vi "GPS data to cluster.vi"(2 "Speed Threshold (km/h)":dbl, 3 "Gps raw data in":string) -> (0 "Arm System?":bool, 1 "GPS Cluster":cluster{"Lat":dbl, "Lon":dbl, "Speed":dbl})   [LabVIEW 2020]
uses:
  <vilib>/express/express arith-compare/Formula/XNode/ExpressFormulaBlockNode.xnode
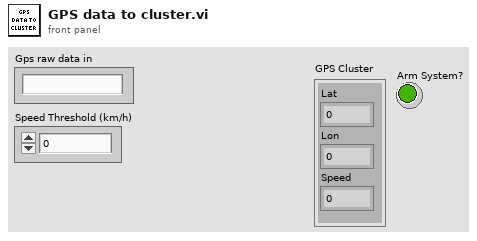
[diagram p1: front panel]
types:
  T1 = typedef "LVDateTimeRec.ctl" = cluster{"fractional second":dbl, "second":i32, "minute":i32, "hour":i32, "day of month":i32, "month":i32, "year":i32, "day of week":i32, "day of year":i32, "DST":i32}
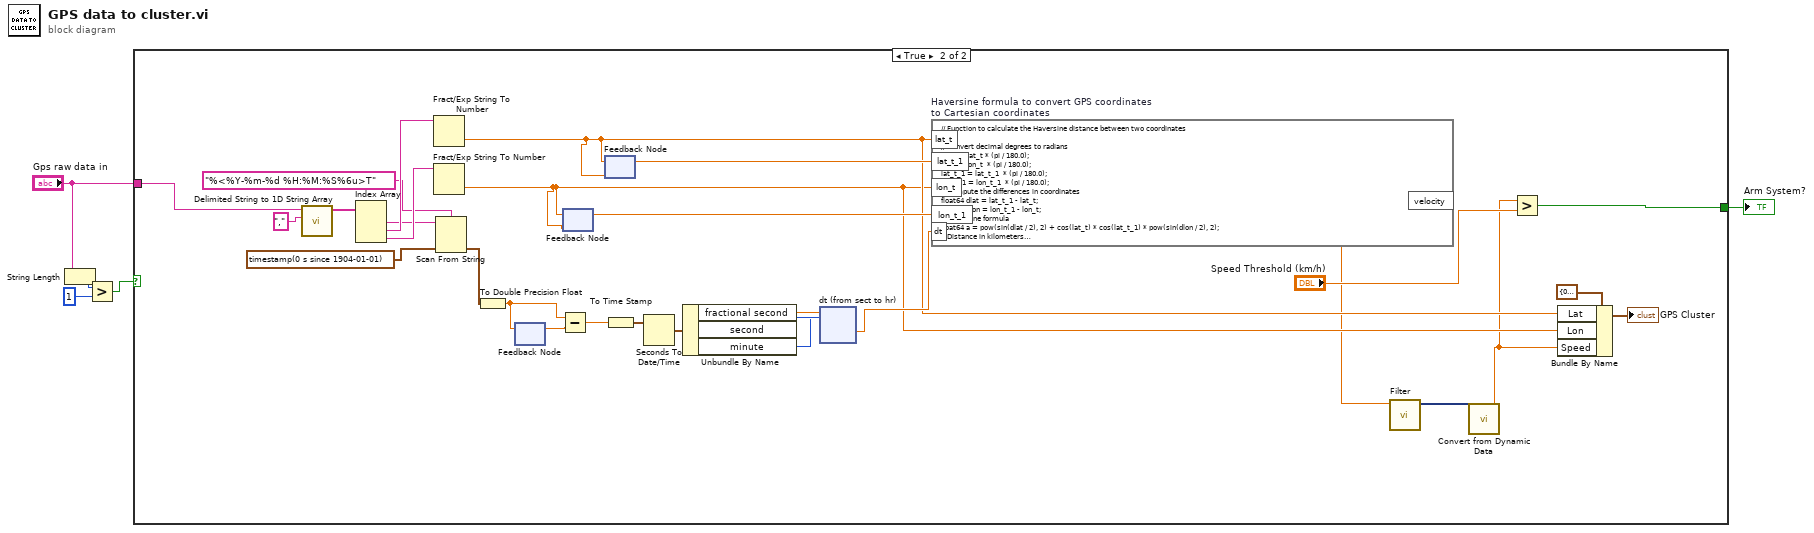
[diagram p0: block diagram]
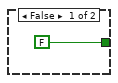
[diagram p2: hidden frame]
diagram:
  n1 = String Length(string="Gps raw data in") -> (length=w2:i32)
  n2 = Greater?(x=w2, y=1) -> (0:w3:bool)
  n3 = case shown="True" w3 {
    tunnel: "Gps raw data in" -> [_ w18]
    tunnel: [FALSE w15] -> w5
    frame False {
    }
    frame True {
      n4 = call <vilib>:"Delimited String to 1D String Array.vi"("delimiter"=",", "delimited string"=w18) -> ("string array"=w34:string[])  [unwired: 9 in]
      n5 = Index Array(array=w34) -> (element #1=w31:string, element #2=w32:string, element #3=w33:string)  [unwired: 3 in]
      n6 = Fract/Exp String To Number(string=w32) -> (number=w11:dbl)  [unwired: 3 in, 1 out]
      n7 = Fract/Exp String To Number(string=w33) -> (number=w10:dbl)  [unwired: 3 in, 1 out]
      n8 = Scan From String(format string="%<%Y-%m-%d %H:%M:%S%6u>T", input string=w31, default 1=timestamp(0 s since 1904-01-01) ("time stamp")) -> (output 1=w26:timestamp)  [unwired: 2 in, 3 out]
      n9 = To Double Precision Float(number=w26) -> (double precision float=w17:dbl)
      n10 = feedback #1() -> (w16:dbl)  [unwired: 1 in]
      n11 = feedback-in #1(w17) -> ()
      n12 = Subtract(x=w17, y=w16) -> (x-y=w27:dbl)
      n13 = feedback #2(w10) -> (w20:dbl)
      n14 = feedback-in #2(w10) -> ()
      n15 = feedback #3(w11) -> (w21:dbl)
      n16 = feedback-in #3(w11) -> ()
      n17 = To Time Stamp(1:w27) -> (0:w28:timestamp)
      n18 = Seconds To Date/Time(time stamp (now)=w28) -> (date time rec=w25:T1)  [unwired: 1 in]
      n19 = Unbundle By Name(w25) -> ("fractional second"=w24:dbl, "second"=w23:i32, "minute"=w22:i32)
      n20 = xnode "dt (from sect to hr)"("X1"=w24, "X2"=w23, "X3"=w22) -> ("Result"=w19:dbl)  [unwired: 1 in, 1 out]
      n21 = formula code="// Function to calculate the Haversine distance between two coordinates\n//\n// Convert decimal degrees to radians\nlat_t = lat_t * (pi / 180.0);\nlon_t =lon_t  * (pi / 180.0);\nlat_t_1 = lat_t_1  * (pi / 180.0);\nlon_t_1 = lon_t_1  * (pi / 180.0);\n// Compute the differences in coordinates\nfloat64 dlat = lat_t_1 - lat_t;\nfloat64 dlon = lon_t_1 - lon_t;\n// Haversine formula\nfloat64 a = pow(sin(dlat / 2), 2) + cos(lat_t) * cos(lat_t_1) * pow(sin(dlon / 2), 2);\n// Distance in kilometers\nfloat EARTH_RADIUS = 6371.0;\nfloat64 Cartesian_distance = EARTH_RADIUS * 2 * atan2(sqrt(a), sqrt(1- a));\nfloat64 velocity = Cartesian_distance / dt;" "Haversine formula to convert GPS coordinates to Cartesian coordinates"("lat_t"=w11, "lat_t_1"=w21, "lon_t"=w10, "lon_t_1"=w20, "dt"=w19) -> ("velocity"=w9:dbl)
      n22 = call "Filter"("Signal"=w9) -> ("Filtered Signal"=w8:dynamicdata)  [unwired: 9 in, 1 out]
      n23 = call "Convert from Dynamic Data"("Dynamic Data Type"=w8) -> ("Scalar"=w7:dbl)  [unwired: 3 in]
      n24 = Greater?(x=w7, y="Speed Threshold (km/h)") -> (0:w15:bool)
      n25 = Bundle By Name(cluster=cluster{"Lat":dbl, "Lon":dbl, "Speed":dbl} {"Lat"=0.0, "Lon"=0.0, "Speed"=0.0} ("GPS"), "Lat"=w11, "Lon"=w10, "Speed"=w7) -> (→"GPS Cluster":cluster{"Lat":dbl, "Lon":dbl, "Speed":dbl})
    }
  }
  "Arm System?" <- w5
